vi "addSpareRows.vi"(0 "reference in":refnum<class "excelFile.lvclass">, 5 "error in (no error)":errorcluster) -> (14 "reference out":refnum<class "excelFile.lvclass">, 19 "error out":errorcluster)   [LabVIEW 2016, in "excelFile.lvclass"]
uses:
  excelFile.lvclass
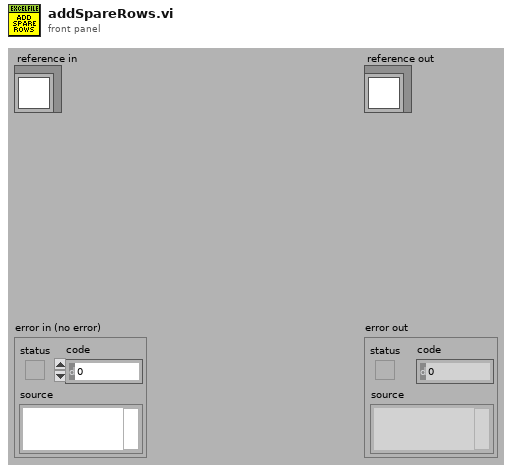
[diagram p1: front panel]
types:
  T1 = typedef "excelFile.lvclass/ObjectAttributesRef.ctl" = refnum<data-value>
  T2 = typedef "excelFile.lvclass/ObjectAttributes.ctl" = cluster{"MyAttribute":dbl, "path":string, "Refnum Excel":cluster{"Excel._Application":refnum<k7>, "Workbooks":refnum<k7>, "Open":refnum<k7>}, "data":string[][][], "save":bool, "fileType":T3, "rowsColor":u32[], "python_ref":refnum<class "python.lvclass">, "items_rows":i32[], "excel_range":i32[][], "TSR":cluster{"number":string, "TSR_path":path, "service_path":path, "email_to":string}, "excel_already_opened?":bool, "file_already_opened?":bool, "excel_protected_opened?":bool, "Refnum Cluster Worksheets":cluster{"Excel._Application":refnum<k7>, "Workbooks":refnum<k7>, "Open":refnum<k7>, "Worksheets":refnum<k7>, "Excel._Worksheet":refnum<k7>}, "#_rows_defective":i32, "#_rows_spare":i32}
  T3 = typedef "excelFile.lvclass/fileType.ctl" = enum16{"devices", "items", "partsTracking", "TSR"}
  T4 = cluster{"Excel._Application":refnum<k7>, "Workbooks":refnum<k7>, "Open":refnum<k7>, "Worksheets":refnum<k7>, "Excel._Worksheet":refnum<k7>}
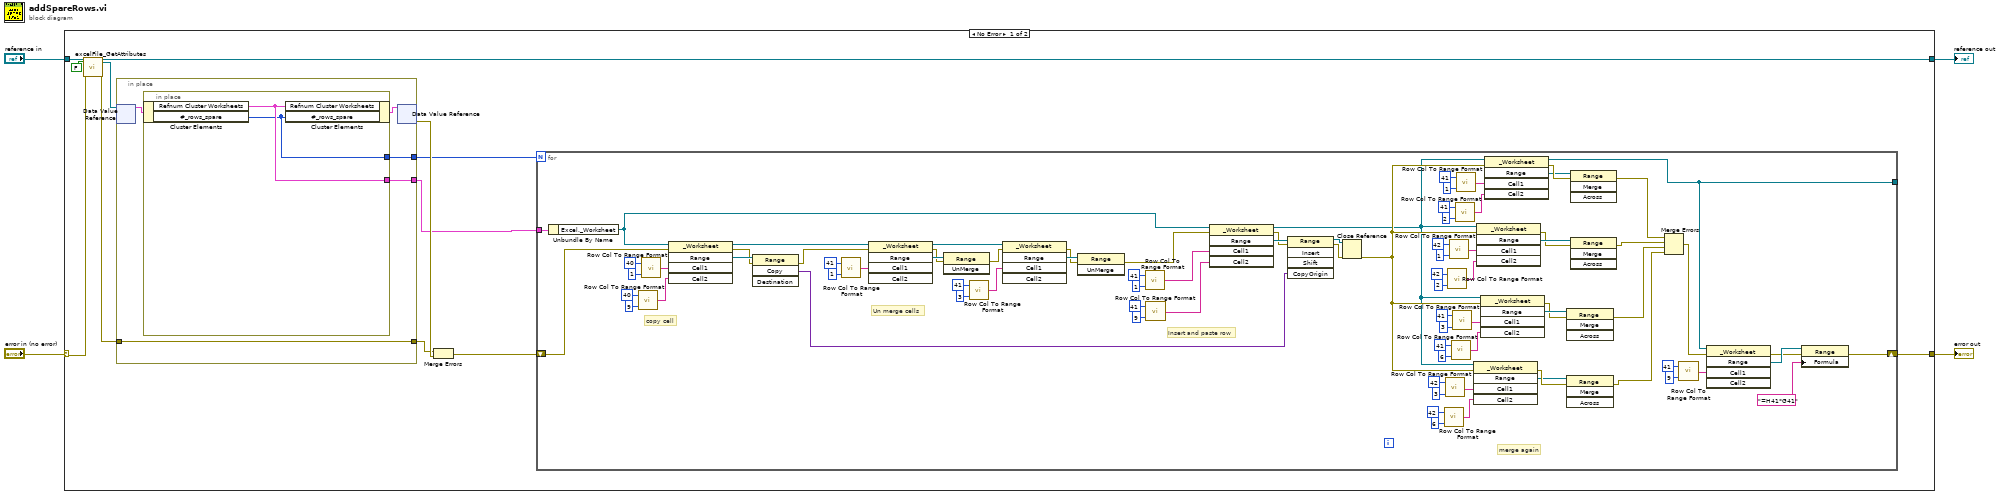
[diagram p0: block diagram]
diagram:
  n1 = case shown="No Error" "error in (no error)" {
    selector: "error in (no error)" -> [w12 w109]
    tunnel: [w7 w109] -> w3
    tunnel: [w10 w108] -> w1
    tunnel: "reference in" -> [w14 w108]
    frame No Error {
      n2 = call "excelFile_GetAttributes.vi"("reference in"=w14, "return data? (T)"=FALSE, "error in (no error)"=w12) -> ("reference out"=w10:refnum<class "excelFile.lvclass">, "attributes ref"=w9:T1, "error out"=w11:errorcluster)  [unwired: 13 in, 1 out]
      n3 = in-place {
        in-place-border: w11 -> [w103]
        in-place-border: [w103] -> w15
        in-place-border: [w102] -> w6
        in-place-border: [w101] -> w5
        n4 = in-place-dvr #1(w9) -> (w104:T2)  [unwired: 1 out]
        n5 = in-place {
          in-place-border: [w107] -> w102
          in-place-border: [w106] -> w101
          n6 = in-place-cluster #2(w104) -> ("Refnum Cluster Worksheets"=w107:T4, "#_rows_spare"=w106:i32)
          n7 = in-place-cluster #2("Refnum Cluster Worksheets"=w107, "#_rows_spare"=w106) -> (w105:T2)
        }
        n8 = in-place-dvr #1(w105) -> (w16:errorcluster)  [unwired: 1 out]
      }
      n9 = Merge Errors(w15, w16) -> (w8:errorcluster)
      n10 = for {
        N: w5 -> [_]
        shift-right: [w18] -> w7
        shift-left: w8 -> [w74]
        tunnel: w6 -> [w64]
        tunnel: [w21] -> _
        # "copy cell"
        # "merge again"
        # "Insert and paste row"
        # "Un merge cells"
        n11 = Unbundle By Name(w64) -> ("Excel._Worksheet"=w73:refnum<k7>)
        n12 = call <userlib>:"Row Col To Range Format.vi"("Column"=9, "Row"=40) -> ("Output String"=w69:string)
        n13 = call <userlib>:"Row Col To Range Format.vi"("Column"=1, "Row"=40) -> ("Output String"=w77:string)
        n14 = invoke class="_Worksheet" method="Range"(reference=w73, error in=w74, "Cell1"=w77, "Cell2"=w69) -> (reference out=w72:refnum<k7>, error out=w67:errorcluster, "Range"=w68:refnum<k7>)  [unwired: 1 in, 2 out]
        n15 = invoke class="Range" method="Copy"(reference=w68, error in=w67) -> (error out=w66:errorcluster, "Copy"=w65:variant)  [unwired: 2 in, 2 out]
        n16 = call <userlib>:"Row Col To Range Format.vi"("Column"=1, "Row"=41) -> ("Output String"=w88:string)
        n17 = invoke class="_Worksheet" method="Range"(reference=w72, error in=w66, "Cell1"=w88) -> (reference out=w82:refnum<k7>, error out=w81:errorcluster, "Range"=w83:refnum<k7>)  [unwired: 2 in, 2 out]
        n18 = invoke class="Range" method="UnMerge"(reference=w83, error in=w81) -> (error out=w80:errorcluster)  [unwired: 1 in, 2 out]
        n19 = call <userlib>:"Row Col To Range Format.vi"("Column"=3, "Row"=41) -> ("Output String"=w85:string)
        n20 = invoke class="_Worksheet" method="Range"(reference=w82, error in=w80, "Cell1"=w85) -> (error out=w79:errorcluster, "Range"=w84:refnum<k7>)  [unwired: 2 in, 3 out]
        n21 = invoke class="Range" method="UnMerge"(reference=w84, error in=w79) -> (error out=w78:errorcluster)  [unwired: 1 in, 2 out]
        n22 = call <userlib>:"Row Col To Range Format.vi"("Column"=1, "Row"=41) -> ("Output String"=w100:string)
        n23 = call <userlib>:"Row Col To Range Format.vi"("Column"=9, "Row"=41) -> ("Output String"=w93:string)
        n24 = invoke class="_Worksheet" method="Range"(reference=w73, error in=w78, "Cell1"=w100, "Cell2"=w93) -> (reference out=w28:refnum<k7>, error out=w91:errorcluster, "Range"=w92:refnum<k7>)  [unwired: 1 in, 2 out]
        n25 = invoke class="Range" method="Insert"(reference=w92, error in=w91, "CopyOrigin"=w65) -> (reference out=w97:refnum<k7>, error out=w96:errorcluster)  [unwired: 2 in, 3 out]
        n26 = Close Reference(reference=w97, error in (no error)=w96) -> (error out=w29:errorcluster)
        n27 = call <userlib>:"Row Col To Range Format.vi"("Column"=6, "Row"=42) -> ("Output String"=w37:string)
        n28 = call <userlib>:"Row Col To Range Format.vi"("Column"=3, "Row"=42) -> ("Output String"=w32:string)
        n29 = call <userlib>:"Row Col To Range Format.vi"("Column"=2, "Row"=42) -> ("Output String"=w56:string)
        n30 = call <userlib>:"Row Col To Range Format.vi"("Column"=1, "Row"=42) -> ("Output String"=w61:string)
        n31 = call <userlib>:"Row Col To Range Format.vi"("Column"=6, "Row"=41) -> ("Output String"=w38:string)
        n32 = call <userlib>:"Row Col To Range Format.vi"("Column"=3, "Row"=41) -> ("Output String"=w42:string)
        n33 = call <userlib>:"Row Col To Range Format.vi"("Column"=2, "Row"=41) -> ("Output String"=w55:string)
        n34 = call <userlib>:"Row Col To Range Format.vi"("Column"=1, "Row"=41) -> ("Output String"=w51:string)
        n35 = invoke class="_Worksheet" method="Range"(reference=w28, error in=w29, "Cell1"=w32, "Cell2"=w37) -> (error out=w34:errorcluster, "Range"=w33:refnum<k7>)  [unwired: 1 in, 3 out]
        n36 = invoke class="_Worksheet" method="Range"(reference=w28, error in=w29, "Cell1"=w61, "Cell2"=w56) -> (error out=w59:errorcluster, "Range"=w60:refnum<k7>)  [unwired: 1 in, 3 out]
        n37 = invoke class="_Worksheet" method="Range"(reference=w28, error in=w29, "Cell1"=w42, "Cell2"=w38) -> (error out=w40:errorcluster, "Range"=w41:refnum<k7>)  [unwired: 1 in, 3 out]
        n38 = invoke class="_Worksheet" method="Range"(reference=w28, error in=w29, "Cell1"=w51, "Cell2"=w55) -> (reference out=w21:refnum<k7>, error out=w53:errorcluster, "Range"=w52:refnum<k7>)  [unwired: 1 in, 2 out]
        n39 = invoke class="Range" method="Merge"(reference=w41, error in=w40) -> (error out=w27:errorcluster)  [unwired: 2 in, 3 out]
        n40 = invoke class="Range" method="Merge"(reference=w33, error in=w34) -> (error out=w26:errorcluster)  [unwired: 2 in, 3 out]
        n41 = invoke class="Range" method="Merge"(reference=w52, error in=w53) -> (error out=w48:errorcluster)  [unwired: 2 in, 3 out]
        n42 = invoke class="Range" method="Merge"(reference=w60, error in=w59) -> (error out=w47:errorcluster)  [unwired: 2 in, 3 out]
        n43 = Merge Errors(w48, w47, w27, w26) -> (w22:errorcluster)
        n44 = call <userlib>:"Row Col To Range Format.vi"("Column"=9, "Row"=41) -> ("Output String"=w25:string)
        n45 = invoke class="_Worksheet" method="Range"(reference=w21, error in=w22, "Cell1"=w25) -> (error out=w19:errorcluster, "Range"=w20:refnum<k7>)  [unwired: 2 in, 3 out]
        n46 = property class="Range"(reference=w20, error in=w19, "Formula"="=H41*G41") -> (error out=w18:errorcluster)  [unwired: 1 out]
      }
    }
    frame Error {
    }
  }
  "error out" <- w3
  "reference out" <- w1
